vi "CLI_PopupPrintParam.vi"(8 "error in (no error)":errorcluster caption="entrée d'erreur (pas d'erreur)", 11 "ParsedParameters":cluster{"Name":string, "Value":string}[](array[cluster])) -> (0 "Error out":errorcluster)   [LabVIEW 2013]
panel:
  out "true":bool
  in  "Ref_Launcher":refnum<vi>
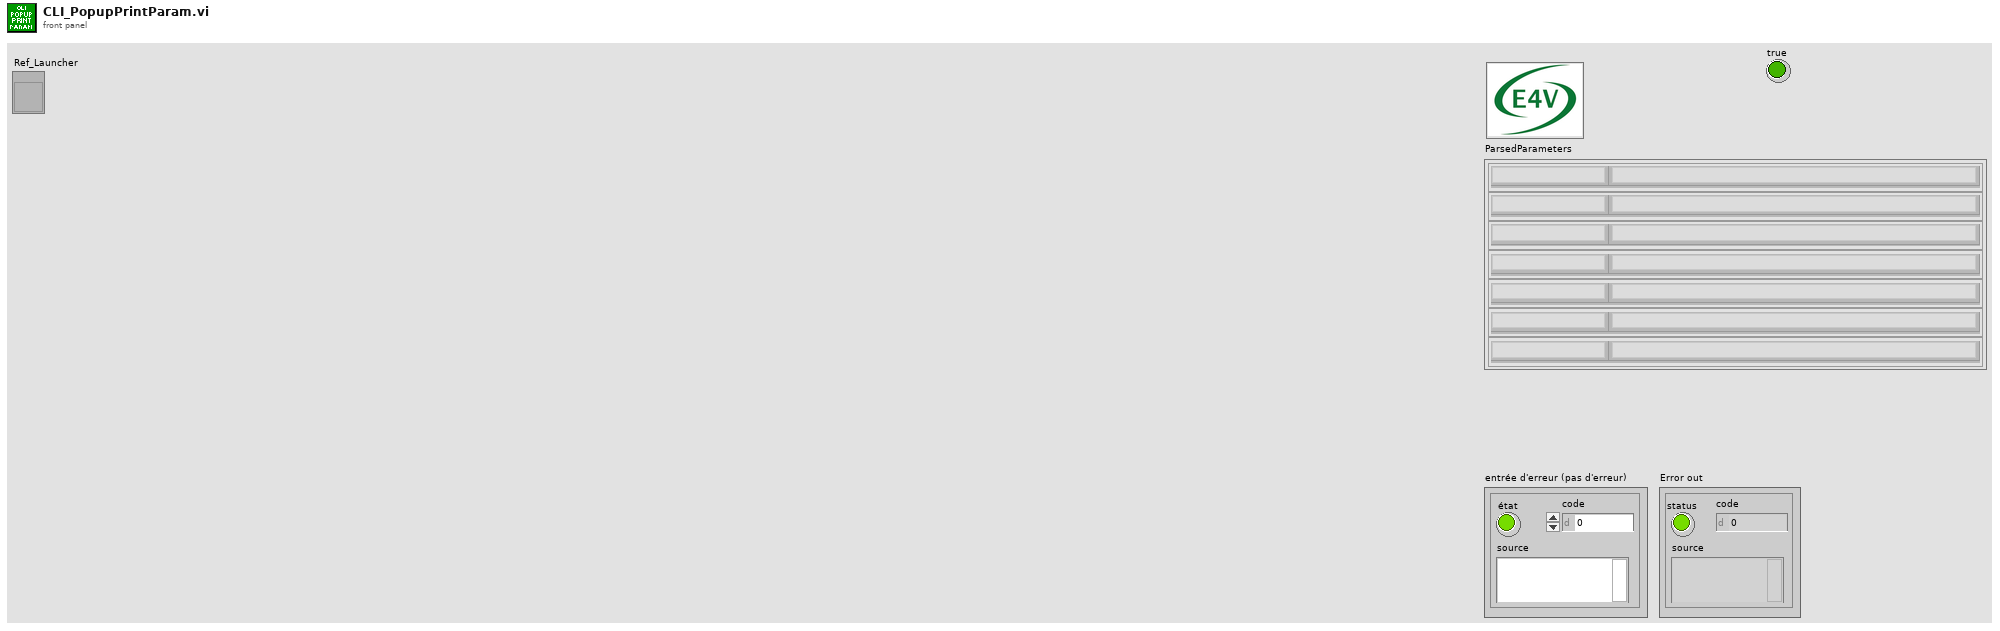
[diagram p1: front panel]
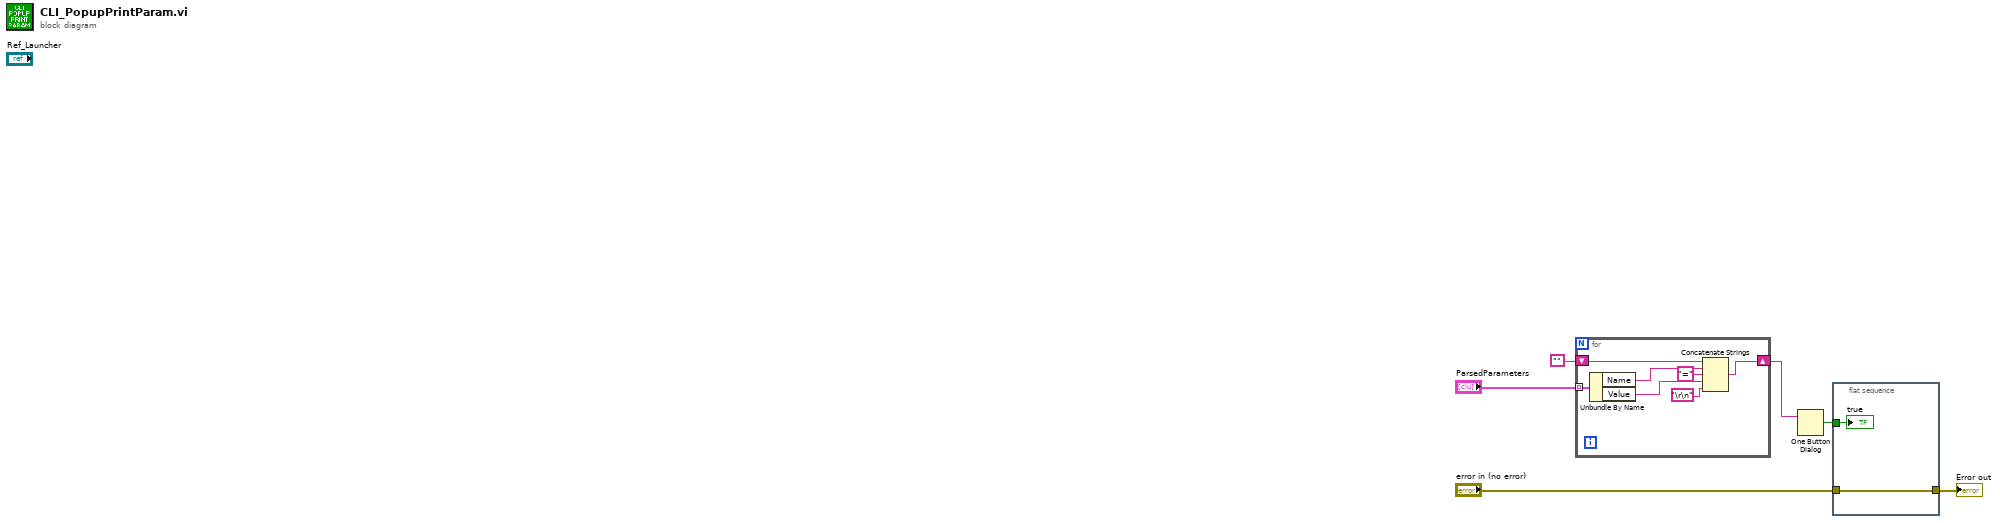
[diagram p0: block diagram]
diagram:
  n1 = for {
    tunnel: "ParsedParameters" -> [w13] mode=indexing
    shift-right: [w7] -> w4
    shift-left: "" -> [w12]
    n2 = Unbundle By Name(w13) -> ("Name"=w11:string, "Value"=w10:string)
    n3 = Concatenate Strings(w12, w11, "=", w10, "\r\n") -> (w7:string)
  }
  n4 = One Button Dialog(message=w4) -> (true=w1:bool)  [unwired: 1 in]
  n5 = flat-sequence {
    tunnel: "error in (no error)" -> [w15]
    tunnel: [w15] -> w2
    tunnel: w1 -> [w14]
    frame #0 {
      "true" <- w14
    }
  }
  "Error out" <- w2
